vi "功能试验判定.vi"(7 "Result":refnum<vi>, 10 "判定参数":T1, 11 "XY曲线":cluster{"X":dbl[], "Y":dbl[]}[](array[cluster])) -> (2 "判定项长度":i32, 3 "OK？":bool)   [LabVIEW 2020]
uses:
  <userlib>/_MGI/1D Array/MGI Average/MGI Average (DBL[]).vi
panel:
  out "逆向平均值":dbl
  out "正向平均值":dbl
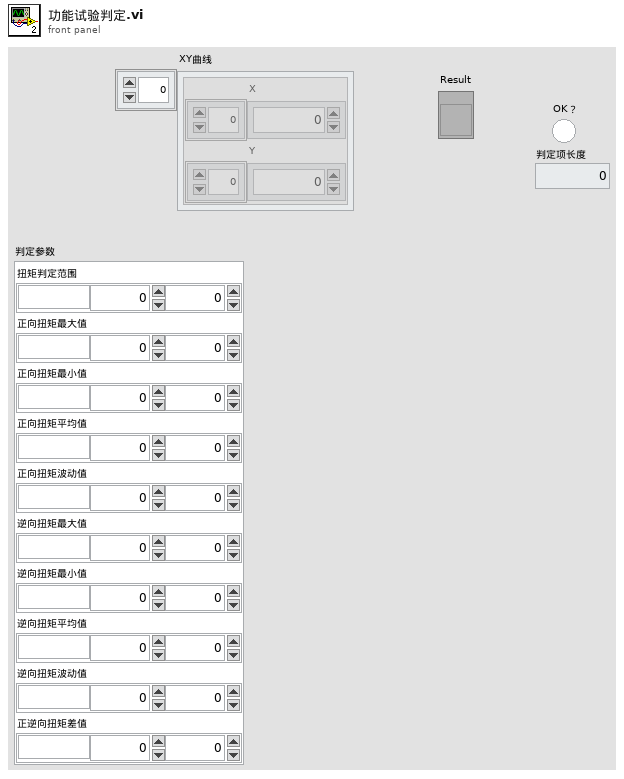
[diagram p1: front panel]
types:
  T1 = cluster{"扭矩判定范围":cluster{"单位":string, "下限":dbl, "上限":dbl}, "正向扭矩最大值":cluster{"单位":string, "下限":dbl, "上限":dbl}, "正向扭矩最小值":cluster{"单位":string, "下限":dbl, "上限":dbl}, "正向扭矩平均值":cluster{"单位":string, "下限":dbl, "上限":dbl}, "正向扭矩波动值":cluster{"单位":string, "下限":dbl, "上限":dbl}, "逆向扭矩最大值":cluster{"单位":string, "下限":dbl, "上限":dbl}, "逆向扭矩最小值":cluster{"单位":string, "下限":dbl, "上限":dbl}, "逆向扭矩平均值":cluster{"单位":string, "下限":dbl, "上限":dbl}, "逆向扭矩波动值":cluster{"单位":string, "下限":dbl, "上限":dbl}, "正逆向扭矩差值":cluster{"单位":string, "下限":dbl, "上限":dbl}}
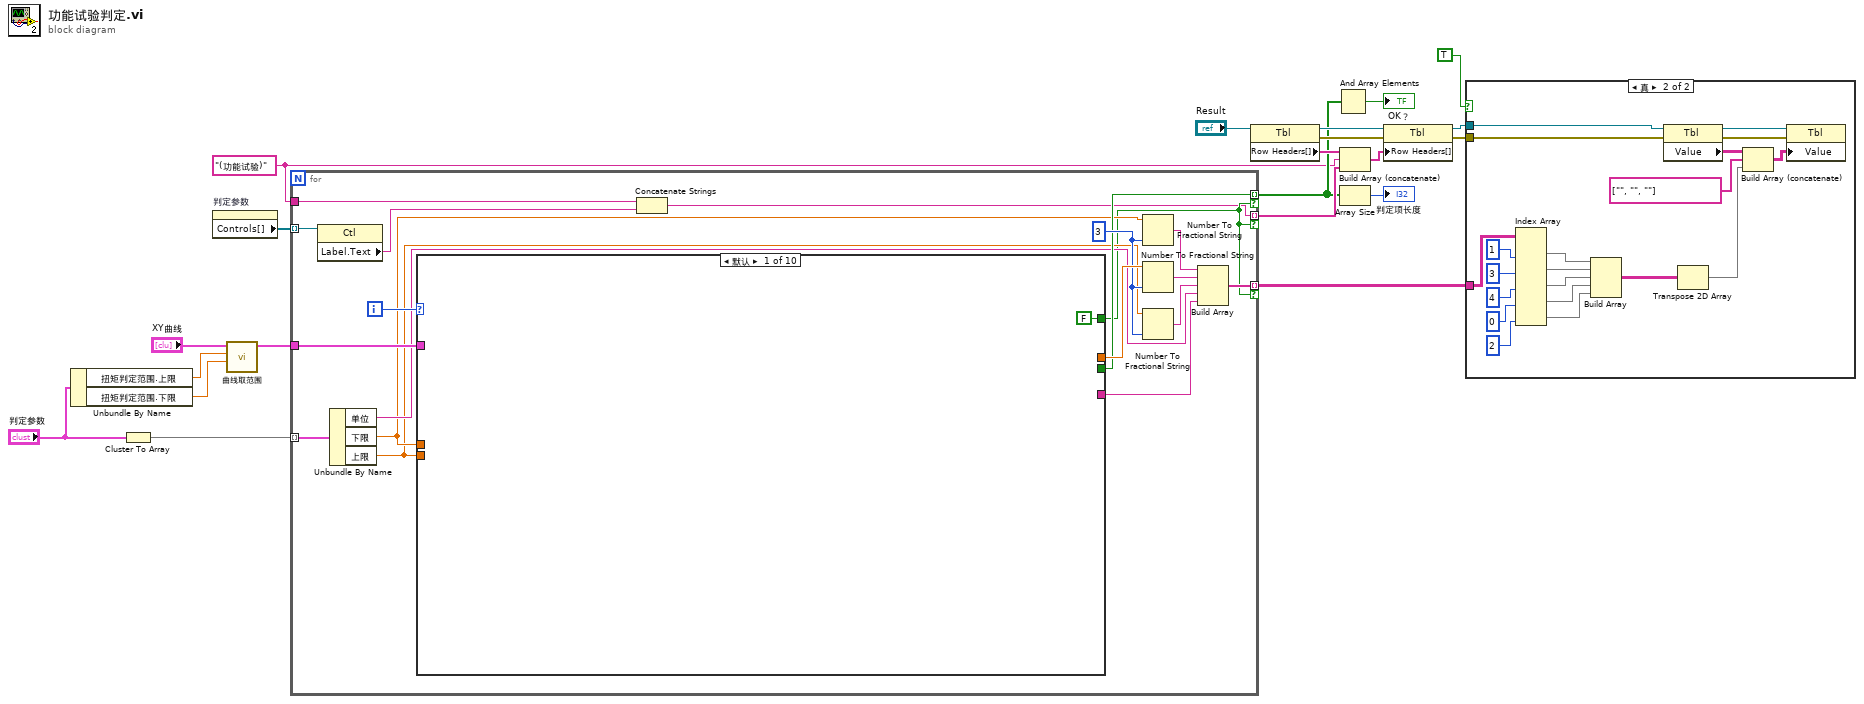
[diagram p0: block diagram]
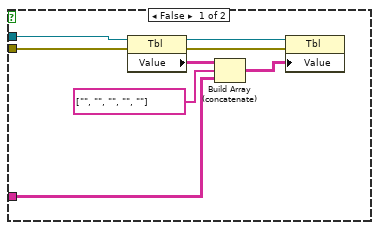
[diagram p2: hidden frame]
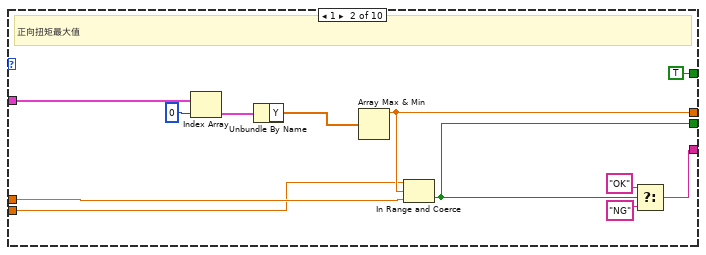
[diagram p3: hidden frame]
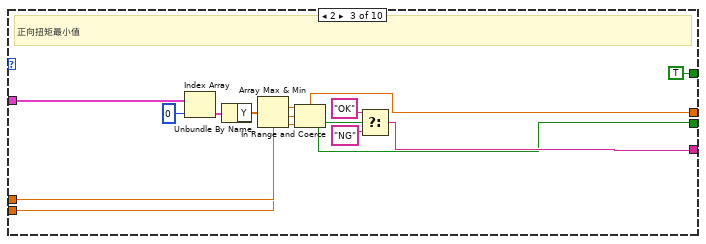
[diagram p4: hidden frame]
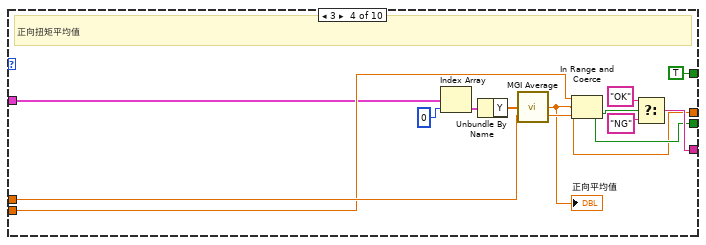
[diagram p5: hidden frame]
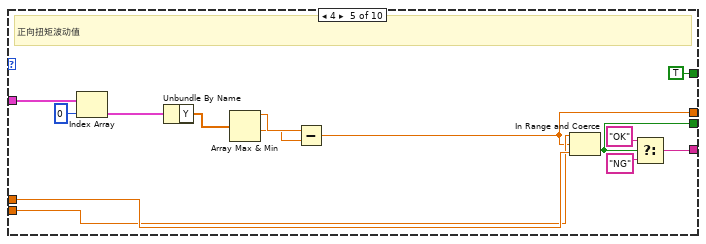
[diagram p6: hidden frame]
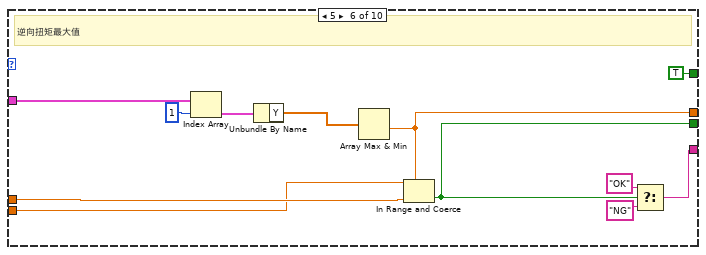
[diagram p7: hidden frame]
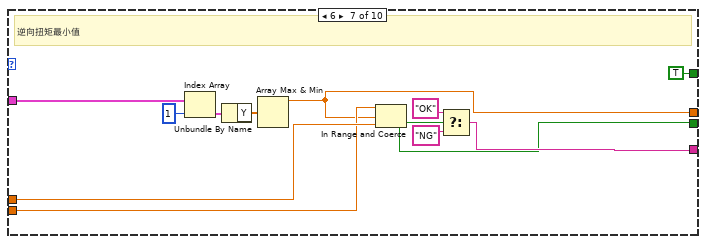
[diagram p8: hidden frame]
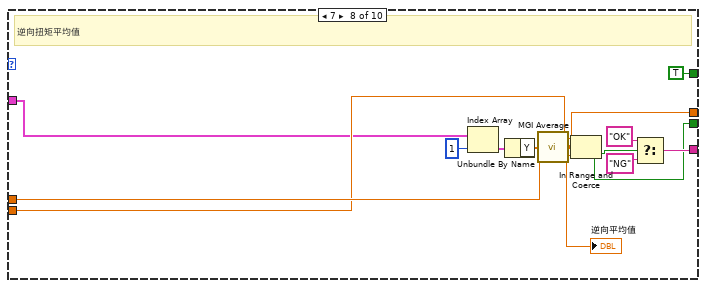
[diagram p9: hidden frame]
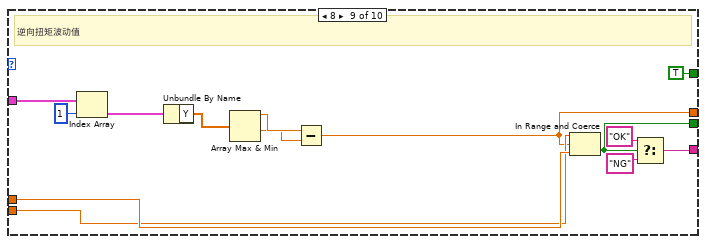
[diagram p10: hidden frame]
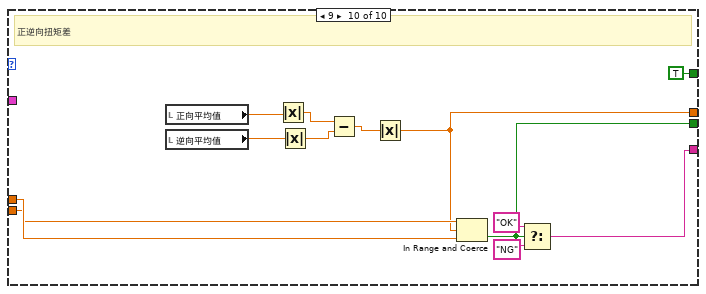
[diagram p11: hidden frame]
diagram:
  w6 = "(功能试验)" ("Label.Text")
  n1 = Unbundle By Name("判定参数") -> ("扭矩判定范围.上限"=w2:dbl, "扭矩判定范围.下限"=w1:dbl)
  n2 = Cluster To Array(cluster="判定参数") -> (array=w21:cluster{"单位":string, "下限":dbl, "上限":dbl}[])
  n3 = property on="判定参数" class="Clust (严格)"() -> ("Controls[]"=w10:refnum<vi>[])  [unwired: 2 in, 2 out]
  n4 = call "曲线取范围.vi"("下限"=w1, "上限"=w2, "曲线In"="XY曲线") -> ("曲线Out"=w4:cluster{"X":dbl[], "Y":dbl[]}[])  [unwired: 8 in]
  n5 = for {
    tunnel: w21 -> [w40] mode=indexing
    tunnel: w10 -> [w38] mode=indexing
    tunnel: w4 -> [w36]
    tunnel: [w30] -> w8 mode=indexing if=w25
    tunnel: [w26] -> w11 mode=indexing if=w25
    tunnel: [w22] -> w14 mode=indexing if=w25
    tunnel: w6 -> [w23]
    i -> [w39]
    w35 = i16 3 ("精度(6)")
    n6 = property class="Ctl"(reference=w38) -> ("Label.Text"=w24:string)  [unwired: 1 in, 2 out]
    n7 = Unbundle By Name(w40) -> ("单位"=w29:string, "下限"=w28:dbl, "上限"=w27:dbl)
    n8 = case shown="默认" w39 {
      tunnel: [_ w50 w56 w66 w78 w92 w104 w116 w128 w142] -> w37
      tunnel: w36 -> [_ w53 w65 w70 w84 w103 w115 w120 w134 _]
      tunnel: [_ w47 w61 w75 w89 w98 w111 w125 w139 w144] -> w31
      tunnel: [_ w46 w60 w74 w88 w97 w110 w124 w138 w143] -> w30
      tunnel: w28 -> [_ w45 w59 w73 w87 w96 w109 w123 w137 w151]
      tunnel: w27 -> [_ w44 w58 w72 w86 w95 w108 w122 w136 w150]
      tunnel: [FALSE TRUE TRUE TRUE TRUE TRUE TRUE TRUE TRUE TRUE] -> w25
      frame Default {
      }
      frame 1 {
        # "正向扭矩最大值"
        n9 = Index Array(array=w53, index=0 ("索引")) -> (element=w51:cluster{"X":dbl[], "Y":dbl[]})
        n10 = Unbundle By Name(w51) -> ("Y"=w42:dbl[])
        n11 = Array Max & Min(array=w42) -> (max value=w50:dbl)  [unwired: 3 out]
        n12 = In Range and Coerce(upper limit=w44, x=w50, lower limit=w45) -> (In Range?=w46:bool)  [unwired: 1 out]
        n13 = Select(t="OK", s=w46, f="NG") -> (s? t:f=w47:string)
      }
      frame 2 {
        # "正向扭矩最小值"
        n14 = Index Array(array=w65, index=0 ("索引")) -> (element=w64:cluster{"X":dbl[], "Y":dbl[]})
        n15 = Unbundle By Name(w64) -> ("Y"=w55:dbl[])
        n16 = Array Max & Min(array=w55) -> (min value=w56:dbl)  [unwired: 3 out]
        n17 = In Range and Coerce(upper limit=w58, x=w56, lower limit=w59) -> (In Range?=w60:bool)  [unwired: 1 out]
        n18 = Select(t="OK", s=w60, f="NG") -> (s? t:f=w61:string)
      }
      frame 3 {
        # "正向扭矩平均值"
        n19 = Index Array(array=w70, index=0 ("索引")) -> (element=w69:cluster{"X":dbl[], "Y":dbl[]})
        n20 = Unbundle By Name(w69) -> ("Y"=w68:dbl[])
        n21 = call-poly <userlib>:"MGI Average.vi"("Double[]"=w68) -> ("Average"=w66:dbl)  [unwired: 1 in]
        "正向平均值" <- w66
        n22 = In Range and Coerce(upper limit=w72, x=w66, lower limit=w73) -> (In Range?=w74:bool)  [unwired: 1 out]
        n23 = Select(t="OK", s=w74, f="NG") -> (s? t:f=w75:string)
      }
      frame 4 {
        # "正向扭矩波动值"
        n24 = Index Array(array=w84, index=0 ("索引")) -> (element=w83:cluster{"X":dbl[], "Y":dbl[]})
        n25 = Unbundle By Name(w83) -> ("Y"=w81:dbl[])
        n26 = Array Max & Min(array=w81) -> (max value=w80:dbl, min value=w79:dbl)  [unwired: 2 out]
        n27 = Subtract(x=w80, y=w79) -> (x-y=w78:dbl)
        n28 = In Range and Coerce(upper limit=w86, x=w78, lower limit=w87) -> (In Range?=w88:bool)  [unwired: 1 out]
        n29 = Select(t="OK", s=w88, f="NG") -> (s? t:f=w89:string)
      }
      frame 5 {
        # "逆向扭矩最大值"
        n30 = Index Array(array=w103, index=1 ("索引")) -> (element=w101:cluster{"X":dbl[], "Y":dbl[]})
        n31 = Unbundle By Name(w101) -> ("Y"=w93:dbl[])
        n32 = Array Max & Min(array=w93) -> (min value=w92:dbl)  [unwired: 3 out]
        n33 = In Range and Coerce(upper limit=w95, x=w92, lower limit=w96) -> (In Range?=w97:bool)  [unwired: 1 out]
        n34 = Select(t="OK", s=w97, f="NG") -> (s? t:f=w98:string)
      }
      frame 6 {
        # "逆向扭矩最小值"
        n35 = Index Array(array=w115, index=1 ("索引")) -> (element=w114:cluster{"X":dbl[], "Y":dbl[]})
        n36 = Unbundle By Name(w114) -> ("Y"=w106:dbl[])
        n37 = Array Max & Min(array=w106) -> (max value=w104:dbl)  [unwired: 3 out]
        n38 = In Range and Coerce(upper limit=w108, x=w104, lower limit=w109) -> (In Range?=w110:bool)  [unwired: 1 out]
        n39 = Select(t="OK", s=w110, f="NG") -> (s? t:f=w111:string)
      }
      frame 7 {
        # "逆向扭矩平均值"
        n40 = Index Array(array=w120, index=1 ("索引")) -> (element=w119:cluster{"X":dbl[], "Y":dbl[]})
        n41 = Unbundle By Name(w119) -> ("Y"=w118:dbl[])
        n42 = call-poly <userlib>:"MGI Average.vi"("Double[]"=w118) -> ("Average"=w116:dbl)  [unwired: 1 in]
        "逆向平均值" <- w116
        n43 = In Range and Coerce(upper limit=w122, x=w116, lower limit=w123) -> (In Range?=w124:bool)  [unwired: 1 out]
        n44 = Select(t="OK", s=w124, f="NG") -> (s? t:f=w125:string)
      }
      frame 8 {
        # "逆向扭矩波动值"
        n45 = Index Array(array=w134, index=1 ("索引")) -> (element=w133:cluster{"X":dbl[], "Y":dbl[]})
        n46 = Unbundle By Name(w133) -> ("Y"=w131:dbl[])
        n47 = Array Max & Min(array=w131) -> (max value=w130:dbl, min value=w129:dbl)  [unwired: 2 out]
        n48 = Subtract(x=w130, y=w129) -> (x-y=w128:dbl)
        n49 = In Range and Coerce(upper limit=w136, x=w128, lower limit=w137) -> (In Range?=w138:bool)  [unwired: 1 out]
        n50 = Select(t="OK", s=w138, f="NG") -> (s? t:f=w139:string)
      }
      frame 9 {
        # "正逆向扭矩差"
        n51 = local read "正向平均值"() -> (w149:dbl)
        n52 = local read "逆向平均值"() -> (w148:dbl)
        n53 = Absolute Value(x=w149) -> (abs(x)=w147:dbl)
        n54 = Absolute Value(x=w148) -> (abs(x)=w146:dbl)
        n55 = Subtract(x=w147, y=w146) -> (x-y=w145:dbl)
        n56 = Absolute Value(x=w145) -> (abs(x)=w142:dbl)
        n57 = In Range and Coerce(upper limit=w150, x=w142, lower limit=w151) -> (In Range?=w143:bool)  [unwired: 1 out]
        n58 = Select(t="OK", s=w143, f="NG") -> (s? t:f=w144:string)
      }
    }
    n59 = Concatenate Strings(w23, w24) -> (w22:string)
    n60 = Number To Fractional String(number=w28, precision (6)=w35) -> (F-format string=w34:string)  [unwired: 2 in]
    n61 = Number To Fractional String(number=w37, precision (6)=w35) -> (F-format string=w33:string)  [unwired: 2 in]
    n62 = Number To Fractional String(number=w27, precision (6)=w35) -> (F-format string=w32:string)  [unwired: 2 in]
    n63 = Build Array(w34, w33, w32, w29, w31) -> (w26:string[])
  }
  n64 = property class="Tbl"(reference="Result") -> (reference out=w16:refnum<vi>, error out=w19:errorcluster, "Row Headers[]"=w12:string[])  [unwired: 1 in]
  n65 = And Array Elements(Boolean array=w8) -> (logical AND=→"OK？":bool)
  n66 = Build Array (concatenate)(w12, w6, w14) -> (w15:string[])
  n67 = Array Size(array=w8) -> (size(s)=→"判定项长度":i32)
  n68 = property class="Tbl"(reference=w16, error in=w19, "Row Headers[]"=w15) -> (reference out=w17:refnum<vi>, error out=w18:errorcluster)
  n69 = case shown="真" TRUE {
    tunnel: w18 -> [w160 w180]
    tunnel: w17 -> [w157 w177]
    tunnel: w11 -> [w156 w168]
    frame False {
      n70 = property class="Tbl"(reference=w157, error in=w160) -> (reference out=w158:refnum<vi>, error out=w159:errorcluster, "Value"=w161:string[][])
      n71 = Build Array (concatenate)(w161, string[] ["", "", "", "", ""], w156) -> (w162:string[][])
      n72 = property class="Tbl"(reference=w158, error in=w159, "Value"=w162) -> ()  [unwired: 2 out]
    }
    frame True {
      n73 = Index Array(array=w168, index (col) #1=1 ("禁用的索引 (列)"), index (col) #2=3 ("索引 (列)"), index (col) #3=4 ("索引 (列)"), index (col) #4=0 ("索引 (列)"), index (col) #5=2 ("索引 (列)")) -> (element #1=w172:string[], element #2=w173:string[], element #3=w174:string[], element #4=w164:string[], element #5=w163:string[])  [unwired: 5 in]
      n74 = Build Array(w172, w173, w174, w164, w163) -> (w175:string[][])
      n75 = property class="Tbl"(reference=w177, error in=w180) -> (reference out=w178:refnum<vi>, error out=w179:errorcluster, "Value"=w181:string[][])
      n76 = Transpose 2D Array(2D array=w175) -> (transposed array=w167:string[][])
      n77 = Build Array (concatenate)(w181, string[] ["", "", ""], w167) -> (w182:string[][])
      n78 = property class="Tbl"(reference=w178, error in=w179, "Value"=w182) -> ()  [unwired: 2 out]
    }
  }
